vi "Sample_Finite_AnlogTrigger.vi"() -> ()   [LabVIEW 2013]
doc: "This samples demonstrates how to sample a finite waveform."
uses:
  <userlib>/ArtScope/Trigger/ArtScope_ConfigureTriggerEdge.vi
  <userlib>/ArtScope/Fetch/ArtScope_FetchBinary8.vi
  <userlib>/ArtScope/_SubVI/ArtScope_ArrayByChannel_U8.vi
panel:
  in  "reference position":dbl
  in  "sensitive":i32=50
  in  "coupling":i32(ring) items=["DC", "AC", "HIG", "LOW"]
  in  "count":i32=1
  in  "slope":i32(ring) items=["Negative", "Positive", "NegatPosit"]
  in  "source":string(combo)="VAL_TRIGGER_ATR"
  in  "level(mV)":dbl=1000.0
  in  "range(Vpp)":i32(ring) items=["20V", "10V", "2V", "40V", "16V", "8V", "4V", "1.6V", "800m", "400m", "160m", "80m", "40m"]
  in  "offset(mV)":i32
  in  "NumSamples":i32=1000
  in  "Stop":bool
  out "waveform":u8[][](graph)
  out "ErrorOutput":errorcluster={"status"=FALSE, "code"=0, "source"="\n"}
  in  "Timeout(s)":dbl=10.0
  in  "MinRecordLength":i32=6000
  in  "MinSampleRate":dbl=800000.0
  in  "Coupling":i32(ring) items=["DC", "AC"]
  in  "Channel Name":string="0"
  in  "Resource Name":string="Dev1"
  # "Vertical"
  # "Horizontal"
  # "Trigger"
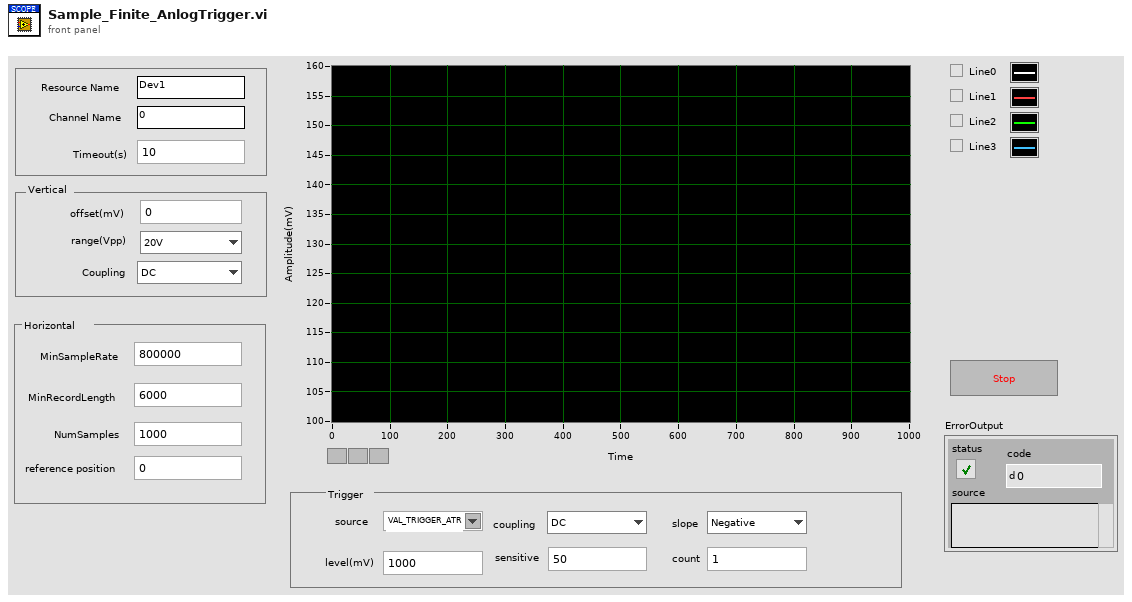
[diagram p1: front panel]
types:
  T1 = cluster{"fLSB":cluster{dbl, dbl, dbl, dbl, dbl, dbl, dbl, dbl}, "RangeValue":cluster{dbl, dbl, dbl, dbl, dbl, dbl, dbl, dbl}, "wMaxLSB":u32, "TriggerMode":i32, "sampLengthPerChan":u32, "pAvailSampsPoints":u32, "channelCount":i32}
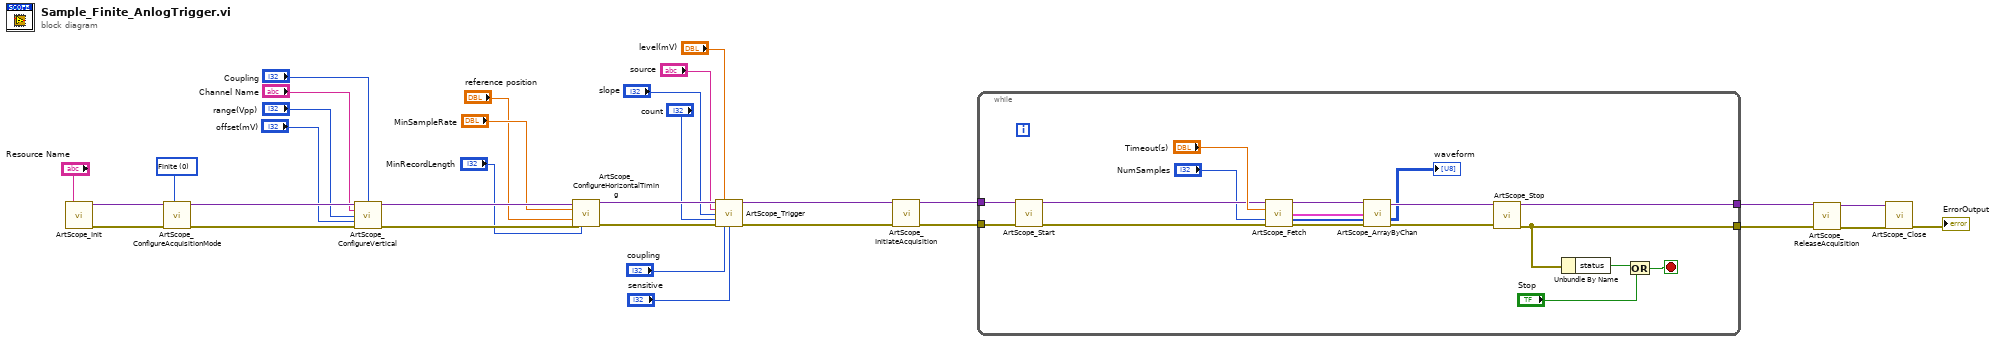
[diagram p0: block diagram]
diagram:
  w24 = 0 items=["Finite", "Continuous"] ("AcuqMode")
  n1 = call <userlib>:"ArtScope_Init.vi"("task name"="Resource Name") -> ("task handle"=w25:variant, "error out"=w26:errorcluster)  [unwired: 13 in]
  n2 = call <userlib>:"ArtScope_ConfigureAcquisitionMode.vi"("task handle"=w25, "acquisition mode"=w24, "error in (no error)"=w26) -> ("task handle"=w23:variant, "error out"=w27:errorcluster)  [unwired: 11 in]
  n3 = call <userlib>:"ArtScope_ConfigureVertical.vi"("task handle"=w23, "coupling"="Coupling", "channels"="Channel Name", "range(Vpp)"="range(Vpp)", "offset"="offset(mV)", "error in (no error)"=w27) -> ("task handle"=w30:variant, "error out"=w29:errorcluster)  [unwired: 8 in]
  n4 = call <userlib>:"ArtScope_ConfigureHorizontalTiming.vi"("task handle"=w30, "min sample rate"="MinSampleRate", "reference position"="reference position", "error in (no error)"=w29, "min record length"="MinRecordLength") -> ("task handle"=w21:variant, "error out"=w22:errorcluster)  [unwired: 9 in]
  n5 = call-poly <userlib>:"ArtScope_Trigger.vi"("task handle"=w21, "level"="level(mV)", "trigger source"="source", "slope"="slope", "trigger count"="count", "error in (no error)"=w22, "trigger coupling"="coupling", "trigger sensitive"="sensitive") -> ("task handle"=w13:variant, "error out"=w12:errorcluster)  [unwired: 6 in]
  n6 = call <userlib>:"ArtScope_InitiateAcquisition.vi"("task handle"=w13, "error in (no error)"=w12) -> ("task handle"=w11:variant, "error out"=w10:errorcluster)  [unwired: 12 in]
  n7 = while {
    tunnel: [w46] -> w17
    tunnel: [w45] -> w16
    tunnel: w11 -> [w44]
    tunnel: w10 -> [w49]
    stop <- w47 stop-if-true
    n8 = call <userlib>:"ArtScope_Start.vi"("task handle"=w44, "error in (no error)"=w49) -> ("task handle"=w42:variant, "error out"=w41:errorcluster)  [unwired: 12 in]
    n9 = call-poly <userlib>:"ArtScope_Fetch.vi"("task handle"=w42, "timeout"="Timeout(s)", "num samples"="NumSamples", "error in (no error)"=w41) -> ("task handle"=w36:variant, "wfm info"=w35:T1, "data"=w34:u8[], "error out"=w39:errorcluster)  [unwired: 8 in]
    n10 = call-poly <userlib>:"ArtScope_ArrayByChan.vi"("task handle"=w36, "wfm info"=w35, "1D data"=w34, "error in (no error)"=w39) -> ("task handle"=w37:variant, "2D data"=→"waveform":u8[][], "error out"=w38:errorcluster)  [unwired: 9 in]
    n11 = call <userlib>:"ArtScope_Stop.vi"("task handle"=w37, "error in (no error)"=w38) -> ("task handle"=w46:variant, "error out"=w45:errorcluster)  [unwired: 12 in]
    n12 = Unbundle By Name(w45) -> ("status"=w48:bool)
    n13 = Or(x=w48, y="Stop") -> (x .or. y?=w47:bool)
  }
  n14 = call <userlib>:"ArtScope_ReleaseAcquisition.vi"("task handle"=w17, "error in (no error)"=w16) -> ("task handle"=w15:variant, "error out"=w14:errorcluster)  [unwired: 12 in]
  n15 = call <userlib>:"ArtScope_Close.vi"("task handle"=w15, "error in (no error)"=w14) -> ("error out"=→"ErrorOutput":errorcluster)  [unwired: 13 in]
